vi "Identify Team from Index.vi"(9 "Players number in":i32=4, 10 "Self index in":i32, 11 "AI Manager in":refnum<class "AI Manager.lvclass">) -> (0 "error out":errorcluster, 3 "AI Manager out":refnum<class "AI Manager.lvclass">)   [LabVIEW 2024, in "AI Manager.lvclass"]
doc: "MIT Licence\nCopyright (c) 2024 David Grollier"
uses:
  AI Manager.lvclass
  AI Manager.lvclass/AI Manager.ctl
  <vilib>/Utility/error.llb/Error Cluster From Error Code.vi
  <vilib>/ErrorRing/Error Ring.xnode
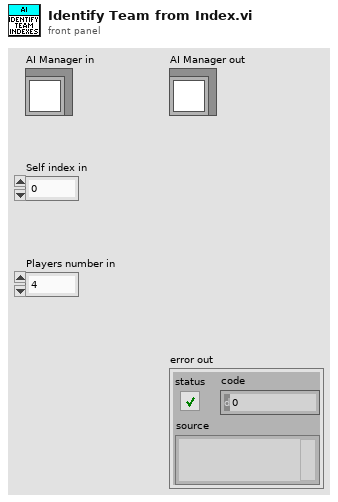
[diagram p1: front panel]
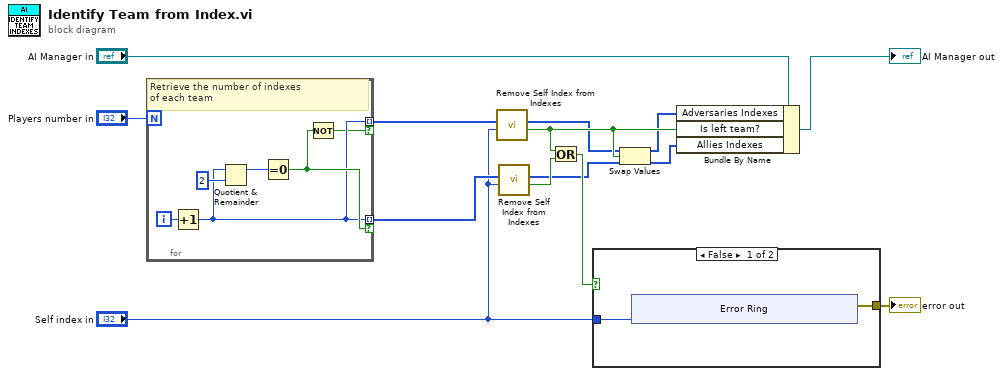
[diagram p0: block diagram]
diagram:
  n1 = for {
    N: "Players number in" -> [_]
    tunnel: [w16] -> w12 mode=indexing if=w17
    tunnel: [w16] -> w10 mode=indexing if=w15
    i -> [w18]
    # "Retrieve the number of indexes\nof each team"
    n2 = Increment(x=w18) -> (x+1=w16:i32)
    n3 = Quotient & Remainder(x=w16, y=2) -> (x-y*floor(x/y)=w19:i32)  [unwired: 1 out]
    n4 = Equal To 0?(x=w19) -> (x = 0?=w17:bool)
    n5 = Not(x=w17) -> (.not. x?=w15:bool)
  }
  n6 = call "Remove Self Index from Indexes.vi"("Self index in"="Self index in", "Indexes in"=w10) -> ("Found?"=w5:bool, "Indexes out"=w4:i32[])  [unwired: 8 in]
  n7 = call "Remove Self Index from Indexes.vi"("Self index in"="Self index in", "Indexes in"=w12) -> ("Found?"=w8:bool, "Indexes out"=w3:i32[])  [unwired: 8 in]
  n8 = Or(x=w5, y=w8) -> (x .or. y?=w9:bool)
  n9 = case shown="False" w9 {
    tunnel: "Self index in" -> [w22 _]
    tunnel: [w21 _] -> w6
    frame False {
      n10 = xnode "Error Ring"("parameter 0"=w22) -> ("error out"=w21:errorcluster)
    }
    frame True {
    }
  }
  "error out" <- w6
  n11 = Swap Values(12:w4, 13:w5, 14:w3) -> (1:w1:i32[], 3:w2:i32[])
  n12 = Bundle By Name(cluster="AI Manager in", "Adversaries Indexes"=w1, "Is left team?"=w5, "Allies Indexes"=w2) -> (→"AI Manager out":refnum<class "AI Manager.lvclass">)
